vi "Read Channel Configuration.vi"(8 "error in (no error)":errorcluster, 11 "Software Lock-in in":refnum<class "Software Lock-in.lvclass">) -> (0 "error out":errorcluster, 3 "Software Lock-in out":refnum<class "Software Lock-in.lvclass">)   [LabVIEW 2016, in "Software Lock-in.lvclass"]
uses:
  Software Lock-in.lvclass
  Software Lock-in.lvclass/Software Lock-in.ctl
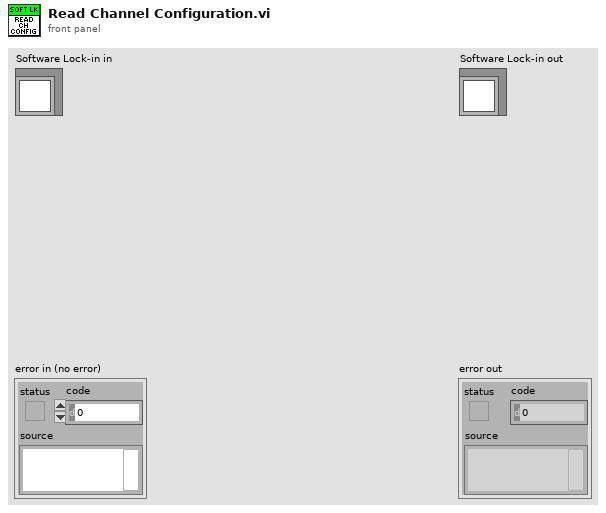
[diagram p1: front panel]
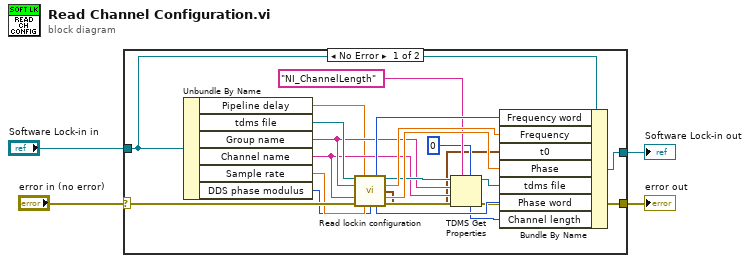
[diagram p0: block diagram]
diagram:
  n1 = case shown="No Error" "error in (no error)" {
    selector: "error in (no error)" -> [w20 w27]
    tunnel: [w15 w27] -> w3
    tunnel: [w23 w26] -> w1
    tunnel: "Software Lock-in in" -> [w25 w26]
    frame No Error {
      n2 = Unbundle By Name(w25) -> ("Pipeline delay"=w9:dbl, "tdms file"=w24:refnum<k34>, "Group name"=w13:string, "Channel name"=w12:string, "Sample rate"=w8:dbl, "DDS phase modulus"=w7:u64)
      n3 = call "Read lockin configuration.vi"("tdms file"=w24, "Pipeline delay"=w9, "group name in"=w13, "Channel name"=w12, "Error In"=w20, "Sample rate"=w8, "DDS phase modulus"=w7) -> ("Frequency word"=w19:u32, "tdms file out"=w14:refnum<k34>, "Frequency"=w22:dbl, "t0"=w5:timestamp, "Phase"=w21:dbl, "Phase word"=w18:u32, "Error Out"=w16:errorcluster)  [unwired: 1 in, 1 out]
      n4 = TDMS Get Properties(5:u64 0, 7:"NI_ChannelLength" ("property name"), 8:w16, 9:w12, 10:w13, 11:w14) -> (0:w15:errorcluster, 3:w10:refnum<k34>, 4:w6:u64)  [unwired: 3 out]
      n5 = Bundle By Name(cluster=w25, "Frequency word"=w19, "Frequency"=w22, "t0"=w5, "Phase"=w21, "tdms file"=w10, "Phase word"=w18, "Channel length"=w6) -> (w23:refnum<class "Software Lock-in.lvclass">)
    }
    frame Error {
    }
  }
  "error out" <- w3
  "Software Lock-in out" <- w1
